vi "Rendezvous Grab Stop.vi"(8 "Error In":errorcluster) -> (0 "Error Out":errorcluster)   [LabVIEW 2019, in "Andor.lvlib"]
uses:
  Andor.lvlib
  Queues/Queues.lvlib
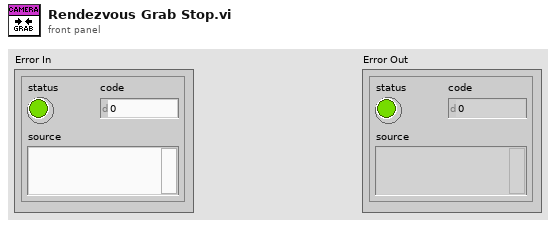
[diagram p1: front panel]
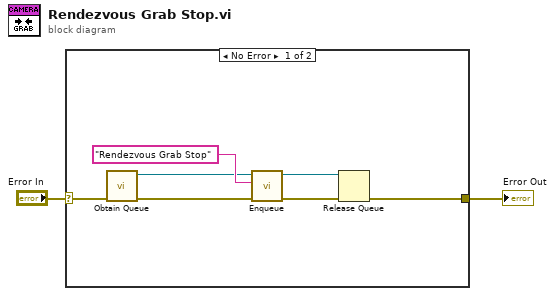
[diagram p0: block diagram]
diagram:
  n1 = case shown="No Error" "Error In" {
    selector: "Error In" -> [w5 w10]
    tunnel: [w6 w10] -> w2
    frame No Error {
      n2 = call "Obtain Queue.vi"("Error In"=w5) -> ("Error Out"=w4:errorcluster, "Queue out"=w3:refnum<queue>)  [unwired: 9 in]
      n3 = call "Enqueue.vi"("Error In"=w4, "State"="Rendezvous Grab Stop", "Queue in"=w3) -> ("Error Out"=w8:errorcluster, "Queue out"=w7:refnum<queue>)  [unwired: 7 in]
      n4 = Release Queue(queue=w7, error in (no error)=w8) -> (error out=w6:errorcluster)  [unwired: 1 in, 2 out]
    }
    frame Error {
    }
  }
  "Error Out" <- w2
